vi "ShiftRegisterUnderstanding.vi"() -> ()   [LabVIEW 2019]
panel:
  out "Output from Current iteration":dbl
  out "Output from 4 iteration ago":dbl
  out "Output from 3 iteration ago":dbl
  out "Output from 2 iteration ago":dbl
  out "OutPut from 1 iteration ago":dbl
  out "Final Output from for Loop":dbl
  out "final Outp[ut for While loop":dbl
  out "Iteration":i32
  in  "stop":bool
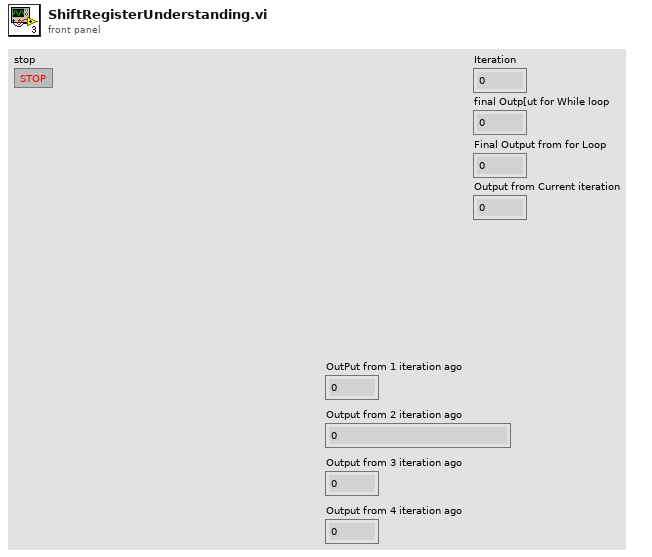
[diagram p1: front panel]
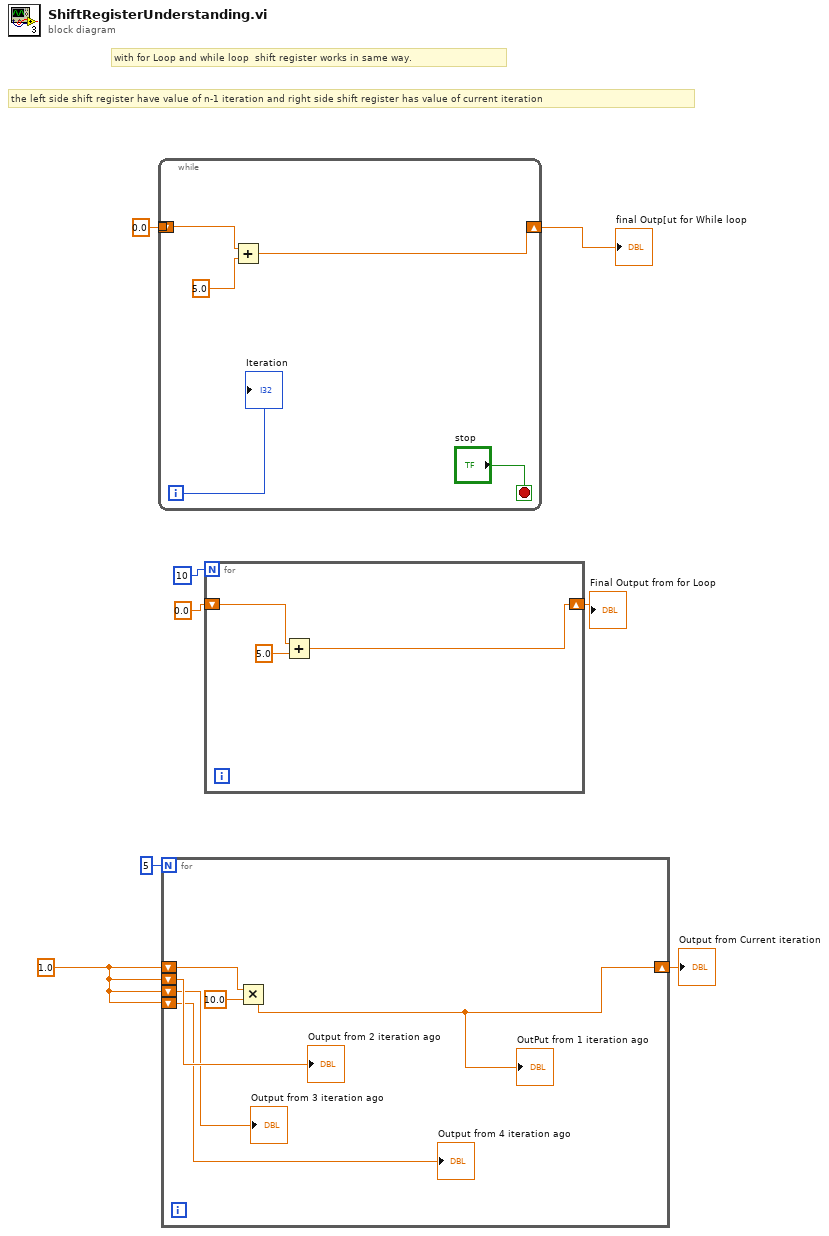
[diagram p0: block diagram]
diagram:
  w2 = 1.0
  # "the left side shift register have value of n-1 iteration and right side shift register has value of current iteration"
  # "with for Loop and while loop  shift register works in same way."
  n1 = while {
    shift-right: [w10] -> w7
    shift-left: 0.0 -> [w9]
    tunnel: [w9] -> _
    i -> [w11]
    stop <- "stop" stop-if-true
    n2 = Add(x=w9, y=5.0) -> (x+y=w10:dbl)
    "Iteration" <- w11
  }
  "final Outp[ut for While loop" <- w7
  n3 = for {
    N: 5 -> [_]
    shift-right: [w17] -> w1
    shift-left: w2 -> [w19]
    shift-left: w2 -> [w16]
    shift-left: w2 -> [w15]
    shift-left: w2 -> [w14]
    n4 = Multiply(x=w19, y=10.0) -> (x*y=w17:dbl)
    "OutPut from 1 iteration ago" <- w17
    "Output from 2 iteration ago" <- w16
    "Output from 3 iteration ago" <- w15
    "Output from 4 iteration ago" <- w14
  }
  "Output from Current iteration" <- w1
  n5 = for {
    N: 10 -> [_]
    shift-right: [w22] -> w4
    shift-left: 0.0 -> [w20]
    n6 = Add(x=w20, y=5.0) -> (x+y=w22:dbl)
  }
  "Final Output from for Loop" <- w4
